vi "WFGStartStopAllCh.vi"(0 "object in":refnum<class "AD2_WFG_SDK.lvclass">, 2 "Start":bool=TRUE, 5 "error in (no error)":errorcluster) -> (14 "object out":refnum<class "AD2_WFG_SDK.lvclass">, 19 "error out":errorcluster)   [LabVIEW 2019, in "AD2_WFG_SDK.lvclass"]
uses:
  AD2_WFG_SDK.lvclass
  AD2_WFG_SDK.lvclass/AD2_WFG_SDK.ctl
  Olasdwf/Olasdwf.lvlib
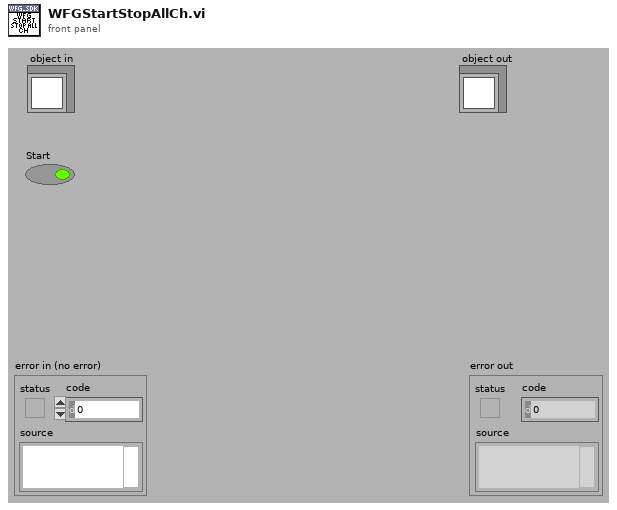
[diagram p1: front panel]
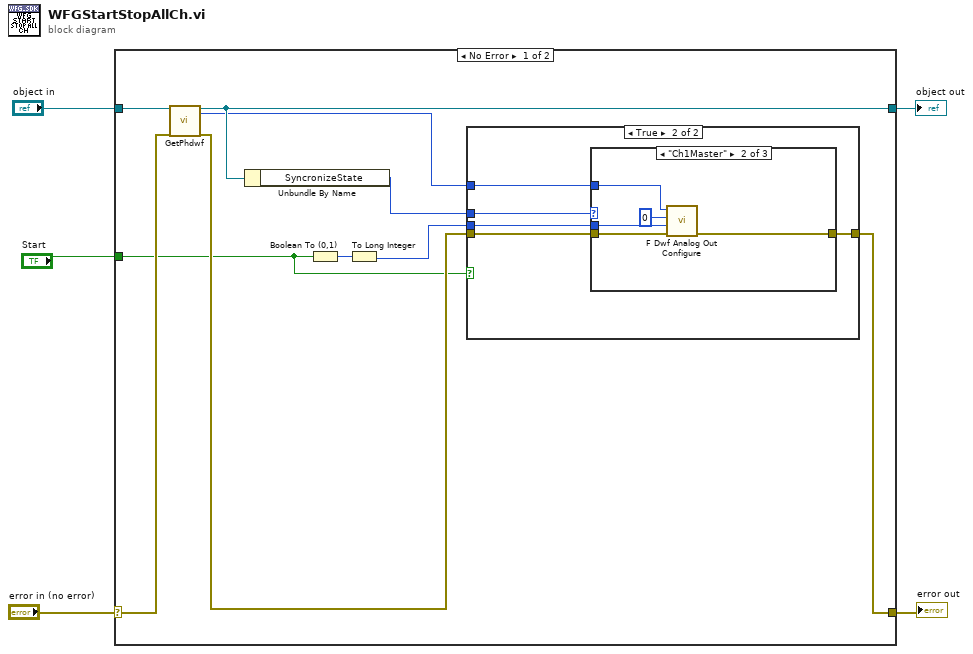
[diagram p0: block diagram]
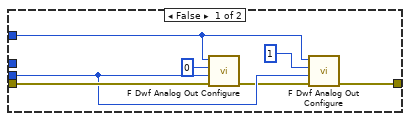
[diagram p2: hidden frame]
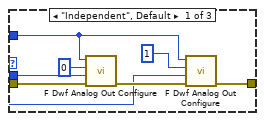
[diagram p3: hidden frame]
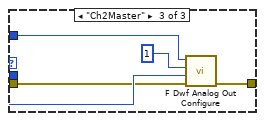
[diagram p4: hidden frame]
diagram:
  n1 = case shown="No Error" "error in (no error)" {
    selector: "error in (no error)" -> [w15 w46]
    tunnel: [w10 w46] -> w4
    tunnel: [w12 w45] -> w2
    tunnel: "object in" -> [w14 w45]
    tunnel: "Start" -> [w6 _]
    frame No Error {
      n2 = call-dynamic "GetPhdwf.vi"("object in"=w14, "error in (no error)"=w15) -> ("object out"=w12:refnum<class "AD2_WFG_SDK.lvclass">, "phdwf"=w8:i32, "error out"=w11:errorcluster)  [unwired: 15 in]
      n3 = Unbundle By Name(w12) -> ("SyncronizeState"=w7:enum16{"Independent", "Ch1Master", "Ch2Master"})
      n4 = Boolean To (0,1)(Boolean=w6) -> (0, 1=w13:i16)
      n5 = To Long Integer(number=w13) -> (32bit integer=w9:i32)
      n6 = case shown="True" w6 {
        tunnel: w11 -> [w22 w27]
        tunnel: [w21 w26] -> w10
        tunnel: w9 -> [w20 w25]
        tunnel: w8 -> [w19 w24]
        tunnel: w7 -> [_ w23]
        frame False {
          n7 = call "F Dwf Analog Out Configure.vi"("error in (no error)"=w22, "fStart"=w20, "idxChannel"=0, "hdwf"=w19) -> ("error out"=w18:errorcluster)  [unwired: 6 in, 1 out]
          n8 = call "F Dwf Analog Out Configure.vi"("error in (no error)"=w18, "fStart"=w20, "idxChannel"=1, "hdwf"=w19) -> ("error out"=w21:errorcluster)  [unwired: 6 in, 1 out]
        }
        frame True {
          n9 = case shown="\"Ch1Master\"" w23 {
            tunnel: w27 -> [w34 w39 w40]
            tunnel: [w32 w35 w44] -> w26
            tunnel: w25 -> [w31 w38 w43]
            tunnel: w24 -> [w28 w36 w41]
            frame "Independent", Default {
              n10 = call "F Dwf Analog Out Configure.vi"("error in (no error)"=w34, "fStart"=w31, "idxChannel"=0, "hdwf"=w28) -> ("error out"=w33:errorcluster)  [unwired: 6 in, 1 out]
              n11 = call "F Dwf Analog Out Configure.vi"("error in (no error)"=w33, "fStart"=w31, "idxChannel"=1, "hdwf"=w28) -> ("error out"=w32:errorcluster)  [unwired: 6 in, 1 out]
            }
            frame "Ch1Master" {
              n12 = call "F Dwf Analog Out Configure.vi"("error in (no error)"=w39, "fStart"=w38, "idxChannel"=0, "hdwf"=w36) -> ("error out"=w35:errorcluster)  [unwired: 6 in, 1 out]
            }
            frame "Ch2Master" {
              n13 = call "F Dwf Analog Out Configure.vi"("error in (no error)"=w40, "fStart"=w43, "idxChannel"=1, "hdwf"=w41) -> ("error out"=w44:errorcluster)  [unwired: 6 in, 1 out]
            }
          }
        }
      }
    }
    frame Error {
    }
  }
  "error out" <- w4
  "object out" <- w2
